vi "Close.vi"(8 "error in (no error)":errorcluster, 11 "NI Fgen in":refnum<class "NI Fgen.lvclass">) -> (0 "error out":errorcluster, 3 "NI Fgen out":refnum<class "NI Fgen.lvclass">)   [LabVIEW 2025, in "Fgen.lvlib" / "NI Fgen.lvclass"]
uses:
  NI Fgen.lvclass
  NI Fgen.lvclass/NI Fgen.ctl
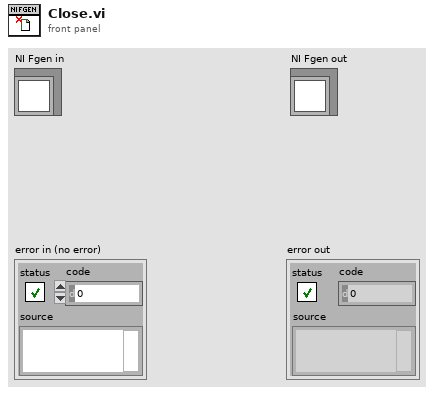
[diagram p1: front panel]
types:
  T1 = typedef "Abstract Engine.lvlibp/Abstract Instrument.lvclass/Channel.ctl" = cluster{"Index":i32, "Alias":string, "Unit":T2, "Upper limit":dbl, "Lower limit":dbl, "Measurement":variant}
  T2 = typedef "Abstract Engine.lvlibp/Abstract Instrument.lvclass/Unit.ctl" = enum16{"V", "A", "Ohm", "Hz", "uF", "degC", "deg"}
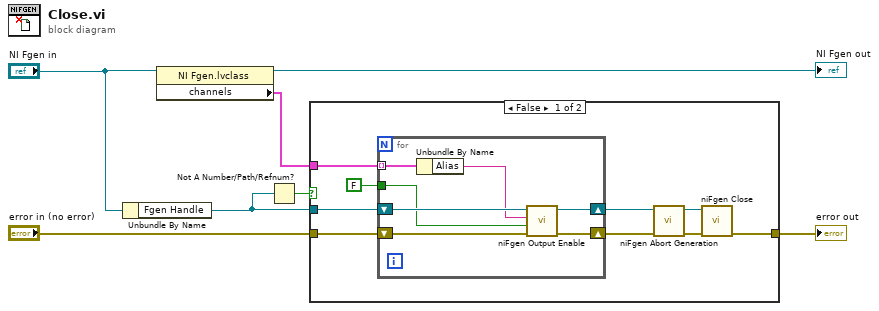
[diagram p0: block diagram]
diagram:
  n1 = Unbundle By Name("NI Fgen in") -> ("Fgen Handle"=w3:refnum<k15>)
  n2 = property class="NI Fgen.lvclass"(reference="NI Fgen in") -> (reference out=→"NI Fgen out":refnum<class "NI Fgen.lvclass">, "channels"=w1:T1[])  [unwired: 1 in, 1 out]
  n3 = Not A Number/Path/Refnum?(number/path/refnum=w3) -> (NaN/Path/Refnum?=w4:bool)
  n4 = case shown="False" w4 {
    tunnel: "error in (no error)" -> [w12 w24]
    tunnel: [w11 w24] -> w5
    tunnel: w3 -> [w10 _]
    tunnel: w1 -> [w9 _]
    frame False {
      n5 = for {
        tunnel: w9 -> [w18] mode=indexing
        shift-right: [w22] -> w13
        shift-left: w12 -> [w21]
        shift-right: [w23] -> w14
        shift-left: w10 -> [w20]
        tunnel: FALSE ("output enable") -> [w19]
        n6 = Unbundle By Name(w18) -> ("Alias"=w17:string)
        n7 = call <instrlib>:"niFgen Output Enable.vi"("error in (no error)"=w21, "Output Enable (default: True)"=w19, "Channel Name"=w17, "Instrument Handle"=w20) -> ("error out"=w22:errorcluster, "Instrument Handle Out"=w23:refnum<k15>)  [unwired: 6 in]
      }
      n8 = call <instrlib>:"niFgen Abort Generation.vi"("error in (no error)"=w13, "Instrument Handle"=w14) -> ("error out"=w16:errorcluster, "Instrument Handle Out"=w15:refnum<k15>)  [unwired: 8 in]
      n9 = call <instrlib>:"niFgen Close.vi"("error in (no error)"=w16, "Instrument Handle"=w15) -> ("error out"=w11:errorcluster)  [unwired: 9 in]
    }
    frame True {
    }
  }
  "error out" <- w5
